vi "External sync mediciones.vi"() -> ()   [LabVIEW 2022 SP3]
doc: "Demonstrates measuring multiple spectra and displaying in a single waveform graph."
uses:
  <vilib>/Utility/file.llb/Write Delimited Spreadsheet (DBL).vi
  20 segundos/Ocean Optics 2000 4000/Ocean Optics 2000 4000.lvlib
panel:
  in  "Tab Control":T1(tab)
  in  "VISA resource name":refnum<visa-resource-name>
  in  "Enable Strobe (Enabled)":bool=TRUE
  in  "Trigger Type (2:External sync)":u8(ring)=2 items=["Normal", "Software Trigger Mode", "External Sync Trigger Mode", "External Hardware Trigger Mode"]
  in  "Si Guardar":bool caption="No Guardar"
  in  "nombre de archivo .txt":string
  in  "Enum":T2(ring)
  in  "Enable Strobe (Disabled)":bool
  out "Numeric":i32
  out "Intensidad":T3(graph)
  in  "stop":bool
  out "psi":cluster{dbl[], dbl[]}(graph)
  out "delta":cluster{dbl[], dbl[]}(graph)
  out "n":cluster{dbl[], dbl[]}(graph)
  out "k":cluster{dbl[], dbl[]}(graph)
  out "e1":cluster{dbl[], dbl[]}(graph)
  out "e2":cluster{dbl[], dbl[]}(graph)
  out "IC 2":cluster{dbl[], dbl[]}(graph)
  out "IS 2":cluster{dbl[], dbl[]}(graph)
  # "(c) 2009-2016 National Instruments.  ALL RIGHTS RESERVED."
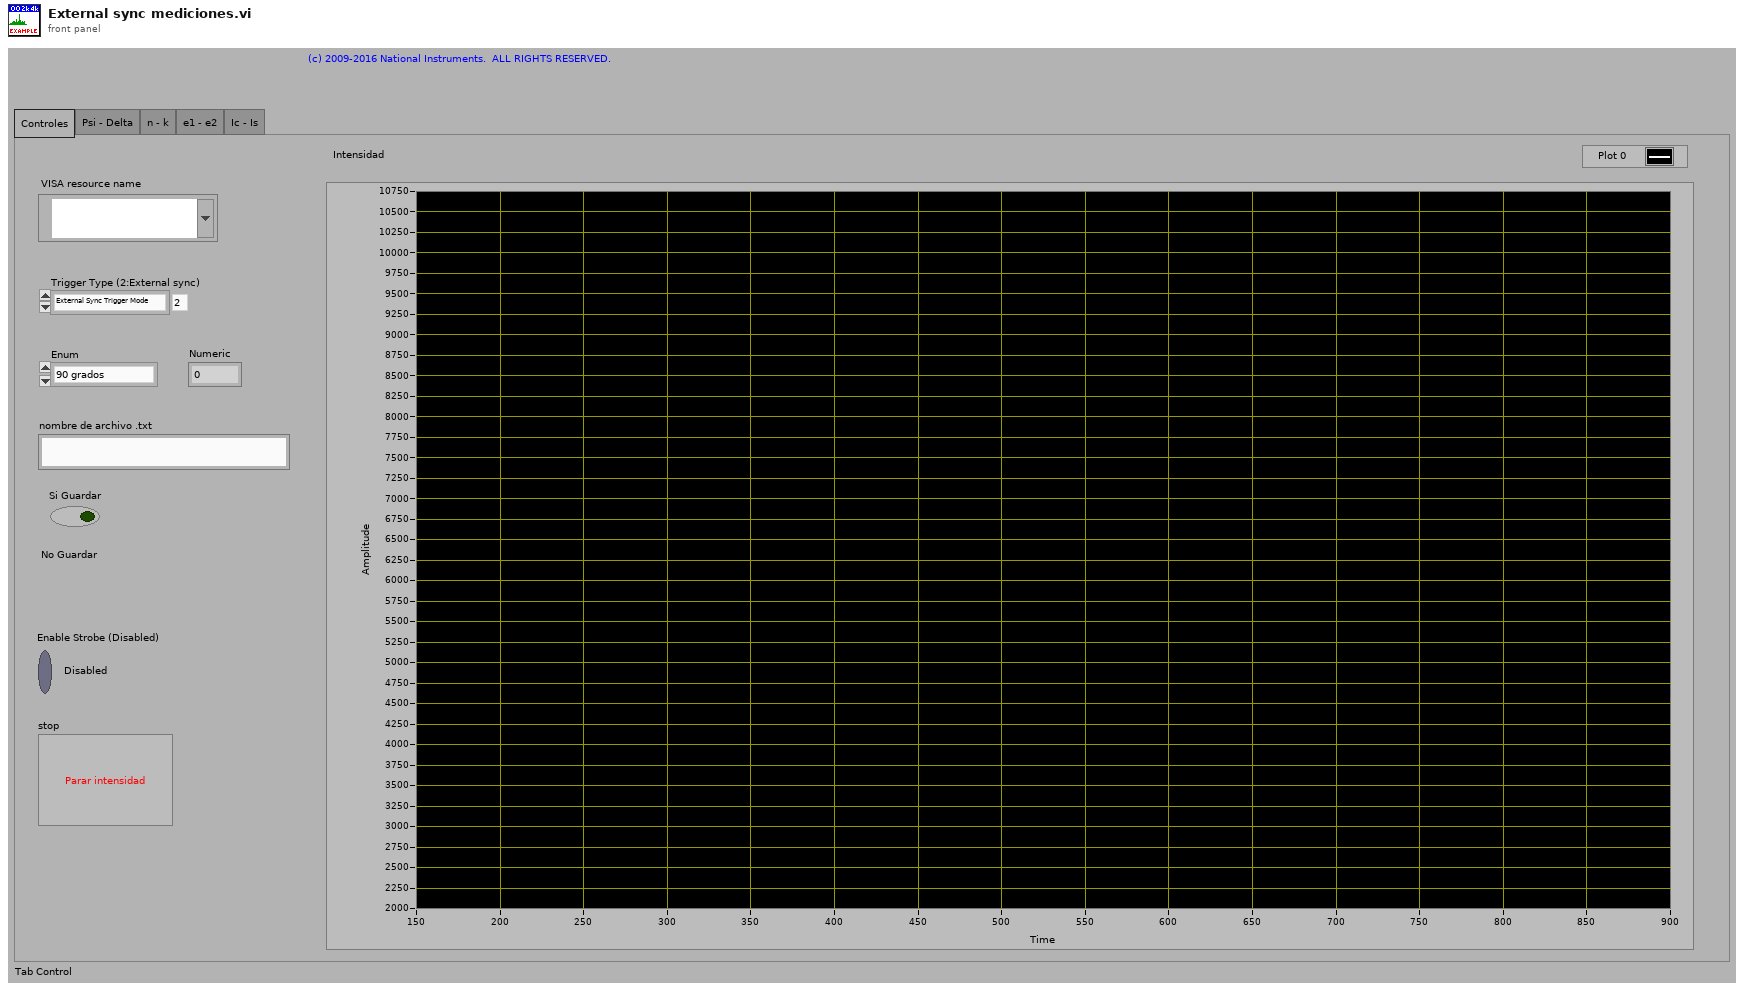
[diagram p1: front panel]
types:
  T1 = enum32{"Controles", "Psi - Delta", "n - k", "e1 - e2", "Ic - Is"}
  T2 = enum16{"90 grados", "180 grados", "360 grados", "FALSE"}
  T3 = cluster{"Wavelength (nm)":dbl[], "Spectrum by Pixel Number":dbl[]}
  T4 = typedef "NI_Matrix.lvlib/RealMatrix.ctl" = dbl[][]
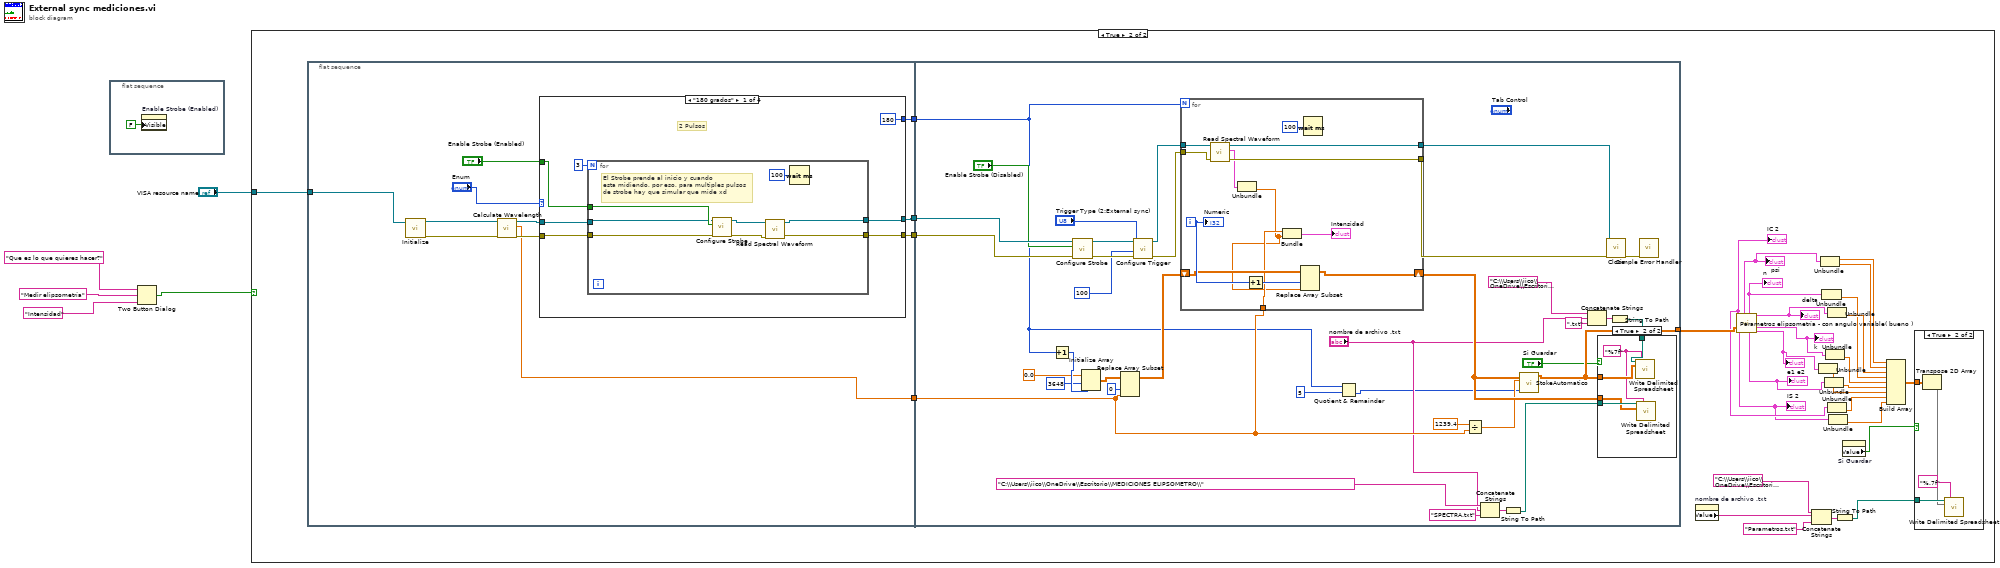
[diagram p0: block diagram]
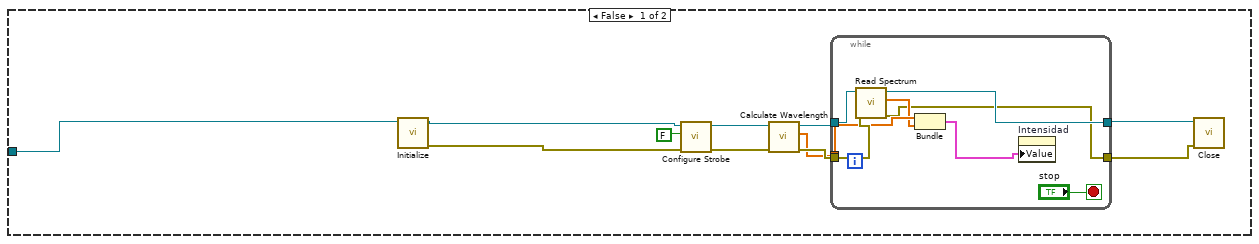
[diagram p2: hidden frame]
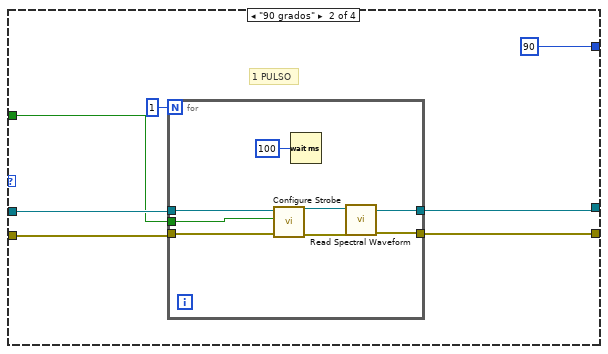
[diagram p4: hidden frame]
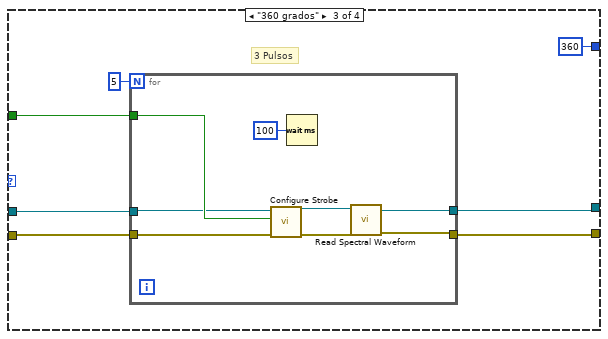
[diagram p5: hidden frame]
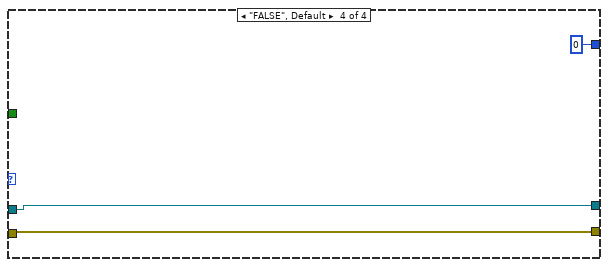
[diagram p6: hidden frame]
diagram:
  n1 = flat-sequence {
    frame #0 {
      n2 = property on="Enable Strobe (Enabled)" class="Bool (strict)"("Visible"=FALSE) -> ()  [unwired: 2 in, 2 out]
    }
  }
  n3 = Two Button Dialog(message="Que es lo que quieres hacer?", 1:"Intensidad" ("F button name (\"Cancel\")"), 2:"Medir elipsometría" ("T button name (\"OK\")")) -> (T button?=w2:bool)
  n4 = case shown="True" w2 {
    tunnel: "VISA resource name" -> [w7 w51]
    frame False {
      n5 = call "Initialize.vi"("VISA resource name"=w7) -> ("error out"=w10:errorcluster, "VISA resource name out"=w11:refnum<visa-resource-name>)  [unwired: 9 in]
      n6 = call "Configure Strobe.vi"("error in (no error)"=w10, "Enable Strobe (Disabled)"=FALSE, "VISA resource name"=w11) -> ("error out"=w16:errorcluster, "VISA resource name out"=w17:refnum<visa-resource-name>)  [unwired: 7 in]
      n7 = call "Calculate Wavelength.vi"("error in (no error)"=w16, "VISA resource name"=w17) -> ("error out"=w13:errorcluster, "Wavelength (nm)"=w12:dbl[], "VISA resource name out"=w14:refnum<visa-resource-name>)  [unwired: 7 in]
      n8 = while {
        tunnel: w12 -> [w23]
        tunnel: w14 -> [w25]
        tunnel: [w21] -> w9
        tunnel: w13 -> [w24]
        tunnel: [w20] -> w8
        stop <- "stop" stop-if-true
        n9 = call "Read Spectrum.vi"("error in (no error)"=w24, "VISA resource name"=w25) -> ("error out"=w20:errorcluster, "Spectrum by Pixel Number"=w22:dbl[], "VISA resource name out"=w21:refnum<visa-resource-name>)  [unwired: 6 in, 1 out]
        n10 = Bundle("Wavelength (nm)"=w23, "Spectrum by Pixel Number"=w22) -> (w19:T3)  [unwired: 1 out]
        n11 = property on="Intensidad" class="XYGraph (strict)"("Value"=w19) -> ()  [unwired: 2 in, 2 out]
      }
      n12 = call "Close.vi"("error in (no error)"=w8, "VISA resource name"=w9) -> ()  [unwired: 9 in, 1 out]
    }
    frame True {
      n13 = flat-sequence {
        tunnel: [w64] -> w55
        tunnel: [w63] -> w54
        tunnel: [w62] -> w53
        tunnel: w51 -> [w61]
        tunnel: [w60] -> w50
        tunnel: w55 -> [w124]
        tunnel: w54 -> [w133]
        tunnel: w53 -> [w132]
        tunnel: [w125] -> w52
        tunnel: w50 -> [w121]
        frame #0 {
          n14 = call "Initialize.vi"("VISA resource name"=w61) -> ("error out"=w70:errorcluster, "VISA resource name out"=w69:refnum<visa-resource-name>)  [unwired: 2 in, 7 out]
          n15 = call "Calculate Wavelength.vi"("error in (no error)"=w70, "VISA resource name"=w69) -> ("error out"=w68:errorcluster, "Wavelength (nm)"=w64:dbl[], "VISA resource name out"=w67:refnum<visa-resource-name>)  [unwired: 7 in]
          n16 = case shown="\"180 grados\"" "Enum" {
            tunnel: w68 -> [w73 w91 w103 w117]
            tunnel: w67 -> [w76 w92 w106 w118]
            tunnel: [w75 w90 w105 w118] -> w63
            tunnel: [w74 w89 w104 w117] -> w62
            tunnel: "Enable Strobe (Enabled)" -> [w72 w88 w102 _]
            tunnel: [180 90 360 0] -> w60
            frame "180 grados" {
              # "2 Pulsos"
              n17 = for {
                N: 3 -> [_]
                tunnel: w76 -> [w83]
                tunnel: [w79] -> w75
                tunnel: [w78] -> w74
                tunnel: w73 -> [w82]
                tunnel: w72 -> [w85]
                # "El Strobe prende al inicio y cuando\nesta midiendo, por eso, para multiples pulsos\nde strobe hay que simular que mide xd"
                n18 = call "Configure Strobe.vi"("error in (no error)"=w82, "Enable Strobe (Disabled)"=w85, "VISA resource name"=w83) -> ("error out"=w80:errorcluster, "VISA resource name out"=w81:refnum<visa-resource-name>)  [unwired: 7 in]
                n19 = call "Read Spectral Waveform.vi"("error in (no error)"=w80, "VISA resource name"=w81) -> ("error out"=w78:errorcluster, "VISA resource name out"=w79:refnum<visa-resource-name>)  [unwired: 7 in, 1 out]
                n20 = Wait (ms)(milliseconds to wait=u32 100) -> ()  [unwired: 1 out]
              }
            }
            frame "90 grados" {
              # "1 PULSO"
              n21 = for {
                N: 1 -> [_]
                tunnel: w88 -> [w98]
                tunnel: w92 -> [w100]
                tunnel: [w94] -> w90
                tunnel: w91 -> [w99]
                tunnel: [w95] -> w89
                n22 = call "Configure Strobe.vi"("error in (no error)"=w99, "Enable Strobe (Disabled)"=w98, "VISA resource name"=w100) -> ("error out"=w96:errorcluster, "VISA resource name out"=w97:refnum<visa-resource-name>)  [unwired: 7 in]
                n23 = Wait (ms)(milliseconds to wait=u32 100) -> ()  [unwired: 1 out]
                n24 = call "Read Spectral Waveform.vi"("error in (no error)"=w96, "VISA resource name"=w97) -> ("error out"=w95:errorcluster, "VISA resource name out"=w94:refnum<visa-resource-name>)  [unwired: 7 in, 1 out]
              }
            }
            frame "360 grados" {
              # "3 Pulsos"
              n25 = for {
                N: 5 -> [_]
                tunnel: w106 -> [w109]
                tunnel: [w111] -> w105
                tunnel: [w112] -> w104
                tunnel: w103 -> [w108]
                tunnel: w102 -> [w114]
                n26 = call "Configure Strobe.vi"("error in (no error)"=w108, "Enable Strobe (Disabled)"=w114, "VISA resource name"=w109) -> ("error out"=w113:errorcluster, "VISA resource name out"=w110:refnum<visa-resource-name>)  [unwired: 7 in]
                n27 = Wait (ms)(milliseconds to wait=u32 100) -> ()  [unwired: 1 out]
                n28 = call "Read Spectral Waveform.vi"("error in (no error)"=w113, "VISA resource name"=w110) -> ("error out"=w112:errorcluster, "VISA resource name out"=w111:refnum<visa-resource-name>)  [unwired: 7 in, 1 out]
              }
            }
            frame "FALSE", Default {
            }
          }
        }
        frame #1 {
          n29 = Increment(x=w121) -> (x+1=w154:i32)
          n30 = call "Configure Strobe.vi"("error in (no error)"=w132, "Enable Strobe (Disabled)"="Enable Strobe (Disabled)", "VISA resource name"=w133) -> ("error out"=w127:errorcluster, "VISA resource name out"=w128:refnum<visa-resource-name>)  [unwired: 7 in]
          n31 = Initialize Array(0.0 ("element"), 3648 ("dimension size"), w154) -> (w137:dbl[][])
          n32 = Replace Array Subset(array=w137, new element=w124, index (col)=0 ("disabled index (col)")) -> (w140:dbl[][])  [unwired: 1 in]
          n33 = call "Configure Trigger.vi"("error in (no error)"=w127, "Hardware Trigger Delay (0 s)"=u16 100, "Trigger Type (0:Normal)"="Trigger Type (2:External sync)", "VISA resource name"=w128) -> ("error out"=w153:errorcluster, "VISA resource name out"=w152:refnum<visa-resource-name>)  [unwired: 6 in]
          n34 = for {
            N: w121 -> [_]
            tunnel: [w172] -> w150
            tunnel: [w171] -> w151
            shift-right: [w167] -> w131
            shift-left: w140 -> [w168]
            tunnel: w152 -> [w166]
            tunnel: w153 -> [w165]
            tunnel: w124 -> [w163]
            i -> [w169]
            n35 = call "Read Spectral Waveform.vi"("error in (no error)"=w165, "VISA resource name"=w166) -> ("error out"=w171:errorcluster, "Spectral Waveform"=w161:cluster{dbl[], dbl[]}, "VISA resource name out"=w172:refnum<visa-resource-name>)  [unwired: 7 out]
            n36 = Unbundle(w161) -> (w160:dbl[])  [unwired: 1 out]
            n37 = Increment(x=w169) -> (x+1=w170:i32)
            n38 = Bundle("Wavelength (nm)"=w163, w160) -> (→"Intensidad":cluster{"Wavelength (nm)":dbl[], dbl[]})  [unwired: 1 in]
            n39 = Replace Array Subset(array=w168, new element=w160, index (col)=w170) -> (w167:dbl[][])  [unwired: 1 in]
            n40 = Wait (ms)(milliseconds to wait=u32 100) -> ()  [unwired: 1 out]
            "Numeric" <- w169
          }
          n41 = Quotient & Remainder(x=w121, y=5) -> (floor(x/y)=w119:i32)  [unwired: 1 out]
          n42 = Divide(x=1239.4, y=w124) -> (x/y=w130:dbl[])
          n43 = Concatenate Strings("C:\\Users\\iico\\OneDrive\\Escritorio\\MEDICIONES ELIPSOMETRO\\", "nombre de archivo .txt", "SPECTRA.txt" ("string")) -> (w148:string)
          n44 = String To Path(string=w148) -> (path=w149:path)
          n45 = call "StokeAutomatico.vi"("# Mediciones / 5"=w119, "Wavelength (nm)"=w130, "Array"=w131) -> ("Real Matrix"=w125:T4)  [unwired: 8 in]
          n46 = Concatenate Strings("C:\\Users\\iico\\OneDrive\\Escritorio\\MEDICIONES ELIPSOMETRO\\", "nombre de archivo .txt", ".txt" ("string")) -> (w142:string)
          n47 = call "Close.vi"("error in (no error)"=w151, "VISA resource name"=w150) -> ("error out"=w134:errorcluster)  [unwired: 9 out]
          n48 = String To Path(string=w142) -> (path=w144:path)
          n49 = case shown="True" "Si Guardar" {
            tunnel: w144 -> [_ w159]
            tunnel: w149 -> [_ w158]
            tunnel: w131 -> [_ w157]
            tunnel: w125 -> [_ w156]
            frame False {
            }
            frame True {
              w155 = "%7f" ("format (%.3f)")
              n50 = call-poly <vilib>:"Write Delimited Spreadsheet.vi"("file path (dialog if empty)"=w159, "format (%.3f)"=w155, "2D data"=w156) -> ()  [unwired: 11 in, 2 out]
              n51 = call-poly <vilib>:"Write Delimited Spreadsheet.vi"("file path (dialog if empty)"=w158, "format (%.3f)"=w155, "2D data"=w157) -> ()  [unwired: 11 in, 2 out]
            }
          }
          n52 = call <vilib>:"Simple Error Handler.vi"("error in (no error)"=w134) -> ()  [unwired: 1 in, 8 out]
        }
      }
      n53 = property on="nombre de archivo .txt" class="Str"() -> ("Value"=w26:string)  [unwired: 2 in, 2 out]
      n54 = call "Parametros elipsometría - con angulo variable( bueno ).vi"("Real Matrix"=w52) -> ("IC 2"=w32:cluster{dbl[], dbl[]}, "psi"=w45:cluster{dbl[], dbl[]}, "n"=w40:cluster{dbl[], dbl[]}, "delta"=w42:cluster{dbl[], dbl[]}, "k"=w38:cluster{dbl[], dbl[]}, "IS 2"=w30:cluster{dbl[], dbl[]}, "e1"=w36:cluster{dbl[], dbl[]}, "e2"=w34:cluster{dbl[], dbl[]})  [unwired: 2 in, 5 out]
      "psi" <- w45
      "delta" <- w42
      "n" <- w40
      "k" <- w38
      "e2" <- w34
      "e1" <- w36
      "IS 2" <- w30
      "IC 2" <- w32
      n55 = Concatenate Strings("C:\\Users\\iico\\OneDrive\\Escritorio\\MEDICIONES ELIPSOMETRO\\", w26, "Parametros.txt" ("string")) -> (w47:string)
      n56 = Unbundle(w34) -> (w33:dbl[])  [unwired: 1 out]
      n57 = Unbundle(w45) -> (w44:dbl[], w43:dbl[])
      n58 = Unbundle(w40) -> (w39:dbl[])  [unwired: 1 out]
      n59 = Unbundle(w36) -> (w35:dbl[])  [unwired: 1 out]
      n60 = Unbundle(w38) -> (w37:dbl[])  [unwired: 1 out]
      n61 = Unbundle(w42) -> (w41:dbl[])  [unwired: 1 out]
      n62 = Unbundle(w32) -> (w31:dbl[])  [unwired: 1 out]
      n63 = Unbundle(w30) -> (w29:dbl[])  [unwired: 1 out]
      n64 = String To Path(string=w47) -> (path=w46:path)
      n65 = property on="Si Guardar" class="Bool (strict)"() -> ("Value"=w27:bool)  [unwired: 2 in, 2 out]
      n66 = Build Array(w44, w43, w41, w39, w37, w35, w33, w31, w29) -> (w28:dbl[][])
      n67 = case shown="True" w27 {
        tunnel: w46 -> [_ w59]
        tunnel: w28 -> [_ w58]
        frame False {
        }
        frame True {
          n68 = Transpose 2D Array(2D array=w58) -> (transposed array=w57:dbl[][])
          n69 = call-poly <vilib>:"Write Delimited Spreadsheet.vi"("file path (dialog if empty)"=w59, "format (%.3f)"="%.7f", "2D data"=w57) -> ()  [unwired: 11 in, 2 out]
        }
      }
    }
  }
